vi "Pre Launch Init.vi"(11 "CS++StartActor in":refnum<class "CS++StartActor.lvclass">) -> (0 "error out":errorcluster, 3 "CS++StartActor out":refnum<class "CS++StartActor.lvclass">)   [LabVIEW 2016, in "CS++StartActor.lvlib" / "CS++StartActor.lvclass"]
doc: "(<B>Filename</B>: Actor Framework.lvlib:Actor.lvclass:Pre Launch Init.vi)\n\nDefines behavior that occurs after the Launch Actor method is invoked but before the actor's Actor Core method begins running.\n\nThe Pre Launch Init method is guaranteed to finish before the Launch Actor method returns to its caller and before the actor itself receives any messages. Any references that the Pre Launch Init method obtains are guaranteed to have the same lifetime as the actor itself. Any errors that the Pre Launch Init method returns will abort the launch.\n\nBy default, this method does nothing. A descendant class may override it to define behavior."
uses:
  CS++StartActor.lvclass
  C:/User/Brand/LVP/CSPP/Packages/CSPP_Core/Actors/CS++BaseActor/CS++BaseActor.lvclass
  CS++BaseActor/CS++BaseActor.lvclass/CS++BaseActor.ctl
  CS++StartActor.lvclass/CS++StartActor.ctl
  Classes/CS++BaseClasses/MessageLogger/CS++MessageLogger.lvclass
  Classes/CS++BaseClasses/Factory/CS++Factory.lvclass
  CS++BaseActor/CS++BaseActor.lvclass
  Libraries/Base/CS++Base.lvlib
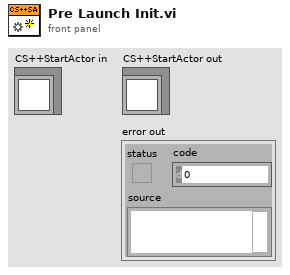
[diagram p1: front panel]
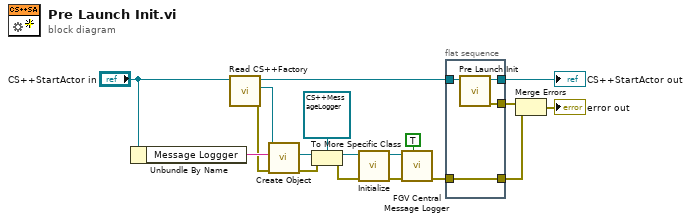
[diagram p0: block diagram]
diagram:
  n1 = Unbundle By Name("CS++StartActor in") -> ("Message Loggger"=w8:string)
  n2 = call "Read CS++Factory.vi"("CS++BaseActor in"="CS++StartActor in") -> ("error out"=w7:errorcluster, "CS++Factory"=w9:refnum<class "CS++Factory.lvclass">, "CS++BaseActor out"=w10:refnum<class "CS++StartActor.lvclass">)  [unwired: 8 in]
  n3 = call "Create Object.vi"("error in (no error)"=w7, "Object Name"=w8, "CS++Factory in"=w9) -> ("error out"=w12:errorcluster, "LabVIEW Object"=w15:refnum<class>)  [unwired: 5 in, 2 out]
  n4 = To More Specific Class(target class=refnum<class "CS++MessageLogger.lvclass"> refnum ("CS++MessageLogger.lvlib:CS++MessageLogger.lvclass"), reference=w15, error in=w12) -> (specific class reference=w6:refnum<class "CS++MessageLogger.lvclass">, error out=w5:errorcluster)
  n5 = call "Initialize.vi"("Error In"=w5, "CS++MessageLogger in"=w6) -> ("Error Out"=w4:errorcluster, "CS++MessageLogger out"=w3:refnum<class "CS++MessageLogger.lvclass">)  [unwired: 8 in]
  n6 = call "FGV Central Message Logger.vi"("Write? (F)"=TRUE ("Write? (f)"), "Error In"=w4, "CS++MessageLogger in"=w3) -> ("Error Out"=w1:errorcluster)  [unwired: 7 in, 1 out]
  n7 = flat-sequence {
    tunnel: [w22] -> w17
    tunnel: [w21] -> w16
    tunnel: w10 -> [w20]
    tunnel: [w19] -> w2
    tunnel: w1 -> [w19]
    frame #0 {
      n8 = call-parent "Pre Launch Init.vi"("CS++BaseActor in"=w20) -> ("error out"=w21:errorcluster, "CS++BaseActor out"=w22:refnum<class "CS++StartActor.lvclass">)  [unwired: 9 in]
    }
  }
  n9 = Merge Errors(w16, w2) -> (→"error out":errorcluster)
  "CS++StartActor out" <- w17
